vi "Test LockinEngine.vi"(8 "error in (no error)":errorcluster, 11 "Lockin.DAQ":refnum<class "Instrument.DAQ.lvclass">) -> (0 "error out":errorcluster, 3 "Lockin.DAQ":refnum<class "Instrument.DAQ.lvclass">)   [LabVIEW 2019, in "Instrument.Lockin.lvlib" / "Instrument.DAQ.lvclass"]
uses:
  Instrument.DAQ.lvclass
  Typedefs/DAQ.Sampling.Sampling--Cluster.ctl
  <vilib>/Analysis/NI_AALBase.lvlib
  <vilib>/Analysis/baseanly.llb/Mean (DBL).vi
  Instrument.Lockin/Instrument.Lockin.lvclass
  Typedefs/Sweep.State--enum.ctl
  Typedefs/AO.Channel.Function--Enum.ctl
  Typedefs/AO.Channel--Cluster--Array.ctl
  Waveguide Model/Waveguide Model--Cluster.ctl
  Typedefs/AO.Channel--Cluster.ctl
  Typedefs/REF.Channel--Cluster.ctl
  Typedefs/REF.Channel--Cluster--Array.ctl
  Instrument.Lockin/Typedefs/Results Type--Enum.ctl
  Typedefs/AI.Channel--Cluster.ctl
  Typedefs/AI.Channel--Cluster--Array.ctl
panel:
  in  "Configuration.AI Channels":T1 {"References" items=["", "1", "2", "3"]; "Channel" min=1}
  in  "Configuration.Channels: REF":T3 {"Roll-Off" min=1; "TC" min=0.0001 format="%#_3p"; "Phase" format="%.3g"; "Frequency" min=0.0001 max=10000.0 format="%.3g"; "Channel" min=1}
  out "refresh rate (Hz)":dbl
  out "Waveform Graph":dbl[][](graph)
  in  "buffer size (samples)":i32
  in  "intervals":i32=10
  out "Histogram Graph":T5(graph)
  in  "sampling":T6={"Fs"=204789.0, "#s"=15753} {"Fs" format="%#_13g"}
  in  "Type":T7
  in  "stop":bool
  in  "Simulate Waveguide":bool
  out "Average time (ms)":dbl=0.328125
  in  "Waveguide Cluster":T8
  out "Waveform Chart 2":u32(graph)
  out "Waveform Chart":dbl[][](graph)=[[-0.22911635604378638]]
  in  "AO Channels":T9=[{"Enable?"=FALSE, "Channel"=0, "Amplitude"=0.0, "Offset"=0.0, "Frequency"=0.1, "Phase"=0.0, "Function"=enum."Sine", "Sweeping?"=FALSE}] {"Phase" format="%.3g"; "Frequency" min=0.0001 max=10000.0 format="%.3g"; "Offset" format="%.3p"; "Amplitude" min=0.0 max=10.0 format="%.3p"}
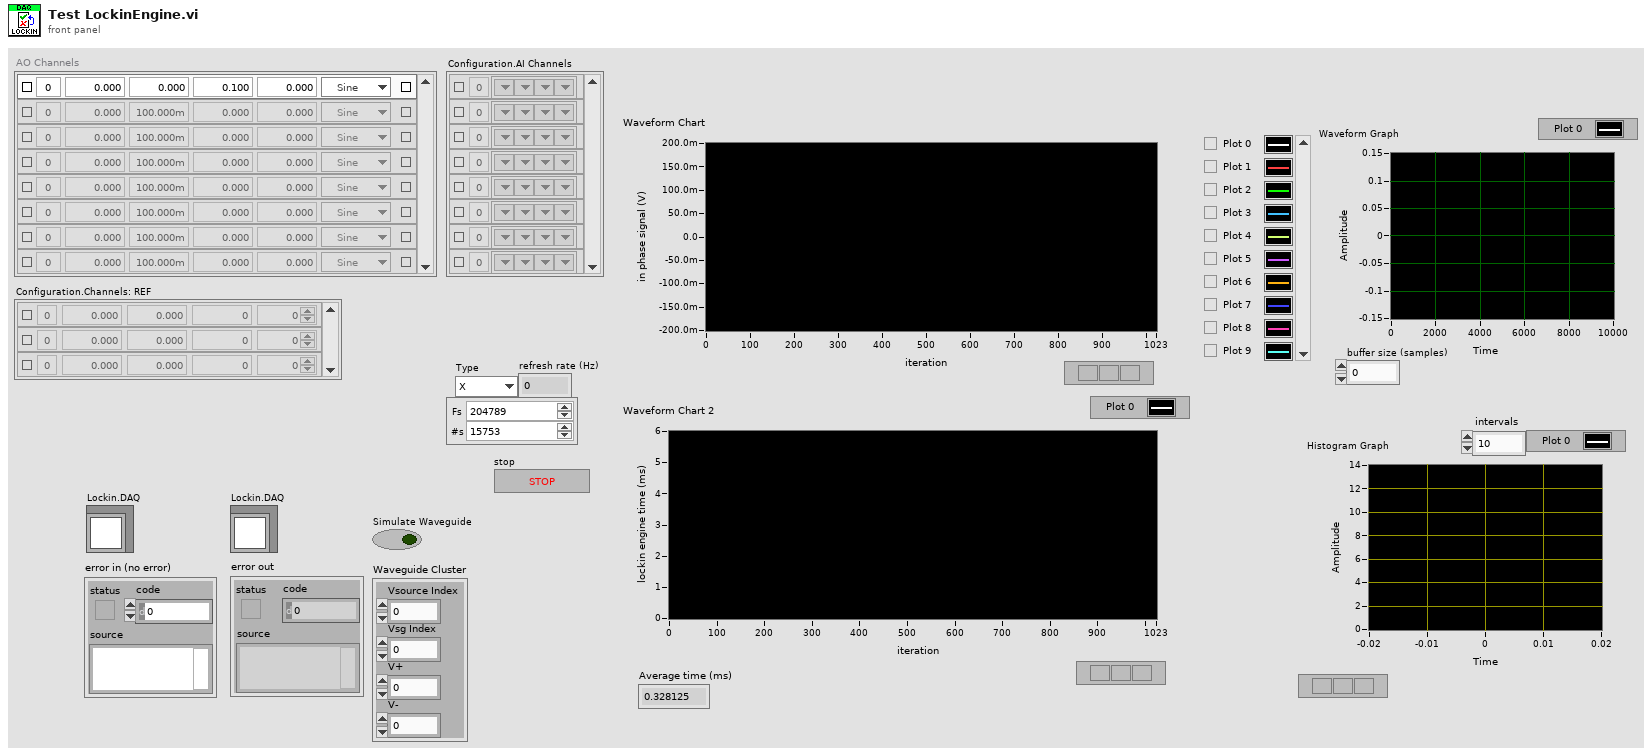
[diagram p1: front panel]
types:
  T1 = typedef "Instrument.Lockin.lvlib/Instrument.DAQ.lvclass/AI.Channel--Cluster--Array.ctl" = T2[]
  T2 = typedef "Instrument.Lockin.lvlib/Instrument.DAQ.lvclass/AI.Channel--Cluster.ctl" = cluster{"Enable?":bool, "Channel":i32, "References":i32[]}
  T3 = typedef "Instrument.Lockin.lvlib/Instrument.DAQ.lvclass/REF.Channel--Cluster--Array.ctl" = T4[]
  T4 = typedef "Instrument.Lockin.lvlib/Instrument.DAQ.lvclass/REF.Channel--Cluster.ctl" = cluster{"Enable?":bool, "Channel":i32, "Frequency":dbl, "Phase":dbl, "TC":dbl, "Roll-Off":i32}
  T5 = cluster{"X Values":dbl[], "Histogram: h(x)":i32[]}[]
  T6 = typedef "Instrument.Lockin.lvlib/Instrument.DAQ.lvclass/DAQ.Sampling.Sampling--Cluster.ctl" = cluster{"Fs":dbl, "#s":i32}
  T7 = typedef "Instrument.Lockin.lvlib/Instrument.Lockin.lvclass/Results Type--Enum.ctl" = enum16{"X", "Y", "R", "Theta", "Mean"}
  T8 = typedef "Instrument.Lockin.lvlib/Instrument.DAQ.lvclass/Waveguide Model--Cluster.ctl" = cluster{"Vsource Index":i32, "Vsg Index":i32, "V+":i32, "V-":i32}
  T9 = typedef "Instrument.Lockin.lvlib/Instrument.DAQ.lvclass/AO.Channel--Cluster--Array.ctl" = T10[]
  T10 = typedef "Instrument.Lockin.lvlib/Instrument.DAQ.lvclass/AO.Channel--Cluster.ctl" = cluster{"Enable?":bool, "Channel":i32, "Amplitude":dbl, "Offset":dbl, "Frequency":dbl, "Phase":dbl, "Function":T11, "Sweeping?":bool}
  T11 = typedef "Instrument.Lockin.lvlib/Instrument.DAQ.lvclass/AO.Channel.Function--Enum.ctl" = enum16{"Sine", "Triangle", "Square"}
  T12 = typedef "Instrument.Lockin.lvlib/Instrument.DAQ.lvclass/Sweep.State--enum.ctl" = enum16{"idle", "initialize", "wait", "sweep", "stop"}
  T13 = typedef "Instrument.Lockin.lvlib/Instrument.DAQ.lvclass/Results--Cluster.ctl" = cluster{"Time Stamp":timestamp, "Results (Dictionary)":cluster{"key":string, "value":dbl}[]}
  T14 = cluster{"X Values":dbl[], "Histogram: h(x)":i32[]}
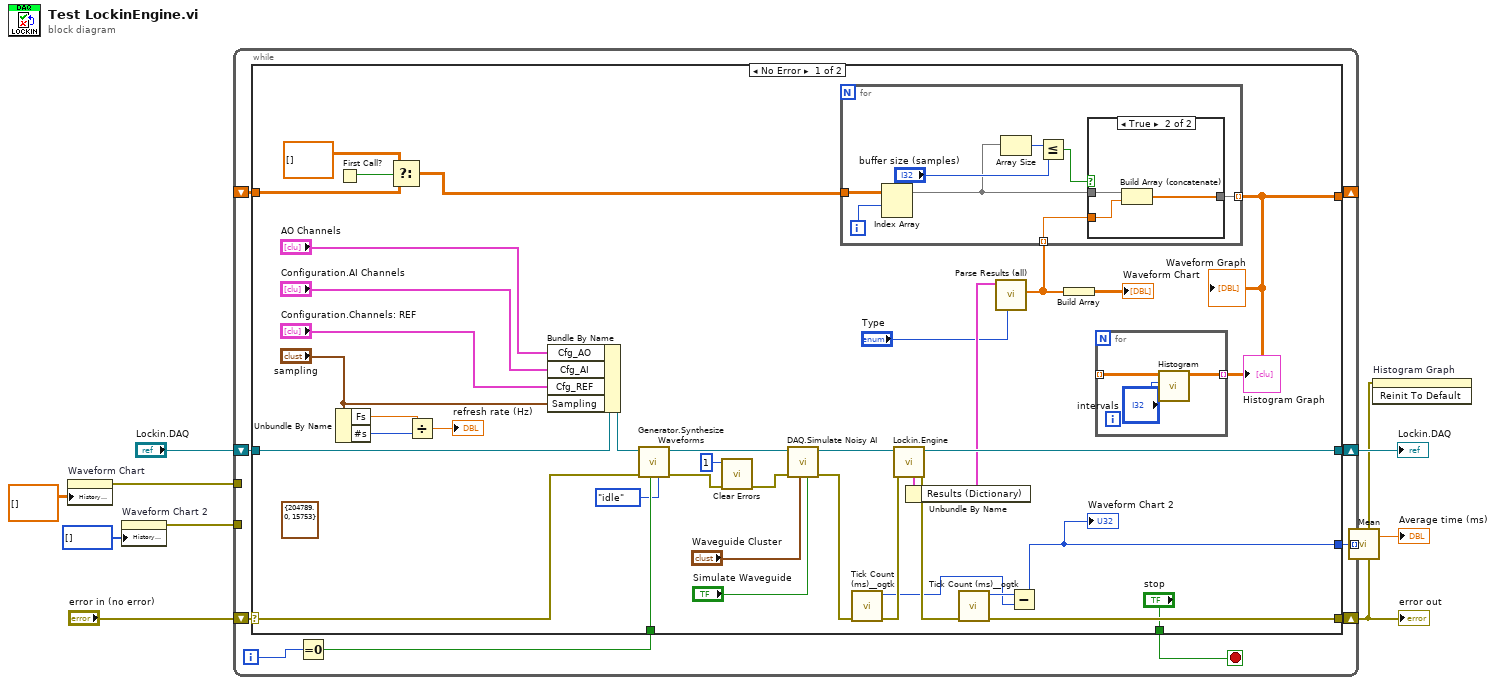
[diagram p0: block diagram]
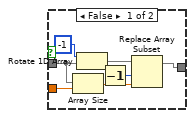
[diagram p2: hidden frame]
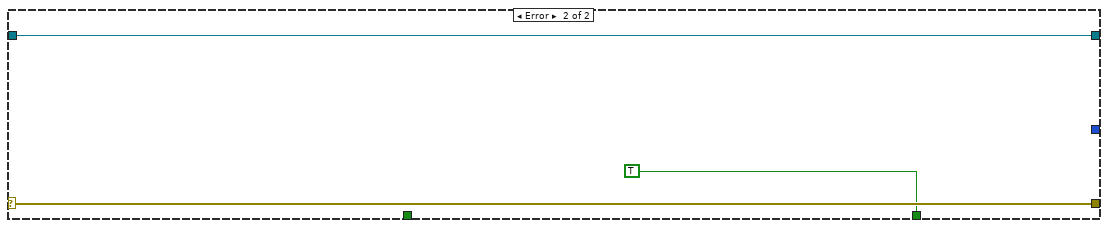
[diagram p3: hidden frame]
diagram:
  n1 = property on="Waveform Chart" class="WFChart (strict)"("History Data"=dbl[][] []) -> (error out=w3:errorcluster)  [unwired: 2 in, 1 out]
  n2 = property on="Waveform Chart 2" class="WFChart (strict)"("History Data"=u32[] []) -> (error out=w4:errorcluster)  [unwired: 2 in, 1 out]
  n3 = while {
    shift-right: [w19] -> w1
    shift-left: "error in (no error)" -> [w20]
    shift-right: [w17] -> w8
    shift-left: "Lockin.DAQ" -> [w18]
    tunnel: [w16] -> w5 mode=indexing
    tunnel: w4 -> [_]
    tunnel: w3 -> [_]
    shift-right: [w12] -> _
    shift-left: _ -> [w11]
    i -> [w14]
    stop <- w13 stop-if-true
    n4 = Equal To 0?(x=w14) -> (x = 0?=w15:bool)
    n5 = case shown="No Error" w20 {
      selector: w20 -> [w58 w83]
      tunnel: [w52 w83] -> w19
      tunnel: [w56 w82] -> w17
      tunnel: w18 -> [w26 w82]
      tunnel: [w50 _] -> w16
      tunnel: w15 -> [w46 _]
      tunnel: ["stop" TRUE ("stop")] -> w13
      tunnel: [w42 _] -> w12
      tunnel: w11 -> [w37 _]
      frame No Error {
        (unwired) T6 {"Fs"=204789.0, "#s"=15753} ("sampling")
        n6 = First Call?() -> (First Call?: T/F=w39:bool)
        n7 = Unbundle By Name("sampling") -> ("Fs"=w36:dbl, "#s"=w35:i32)
        n8 = Select(t=dbl[][] [], s=w39, f=w37) -> (s? t:f=w38:dbl[][])
        n9 = Divide(x=w36, y=w35) -> (x/y=→"refresh rate (Hz)":dbl)
        n10 = Bundle By Name(cluster=w26, "Cfg_AO"="AO Channels", "Cfg_AI"="Configuration.AI Channels", "Cfg_REF"="Configuration.Channels: REF", "Sampling"="sampling") -> (w28:refnum<class "Instrument.DAQ.lvclass">)
        n11 = call "Generator.Synthesize Waveforms.vi"("sweep state"=Sweep.State--enum."idle", "Reset Phase?"=w46, "error in (no error)"=w58, "Instrument.DAQ"=w28) -> ("error out"=w24:errorcluster, "Instrument.DAQ"=w59:refnum<class "Instrument.DAQ.lvclass">)  [unwired: 6 in]
        n12 = call <vilib>:"Clear Errors.vi"("error in (no error)"=w24, "specific error code to clear (0: all)"=1) -> ("error out"=w23:errorcluster)  [unwired: 4 in, 1 out]
        n13 = call "DAQ.Simulate Noisy AI.vi"("Simulate Waveguide [T]"="Simulate Waveguide", "Waveguide Cluster"="Waveguide Cluster", "error in (no error)"=w23, "Instrument.DAQ in"=w59) -> ("error out"=w54:errorcluster, "Instrument.DAQ out"=w57:refnum<class "Instrument.DAQ.lvclass">)  [unwired: 6 in]
        n14 = call <userlib>:"Tick Count (ms)__ogtk.vi"("error in (no error)"=w54) -> ("error out"=w53:errorcluster, "millisecond timer value"=w43:u32)  [unwired: 9 in]
        n15 = call "Lockin.Engine.vi"("error in (no error)"=w53, "Instrument.DAQ"=w57) -> ("error out"=w49:errorcluster, "<Results> (X,Y,R,Theta,Mean)"=w55:T13, "Instrument.DAQ out"=w56:refnum<class "Instrument.DAQ.lvclass">)  [unwired: 7 in]
        n16 = Unbundle By Name(w55) -> ("Results (Dictionary)"=w33:cluster{"key":string, "value":dbl}[])
        n17 = call <userlib>:"Tick Count (ms)__ogtk.vi"("error in (no error)"=w49) -> ("error out"=w52:errorcluster, "millisecond timer value"=w51:u32)  [unwired: 9 in]
        n18 = call "Parse Results (all).vi"("Type"="Type", "Results (Dictionary)"=w33) -> ("Data"=w32:dbl[])  [unwired: 6 in, 3 out]
        n19 = for {
          tunnel: w38 -> [w70]
          tunnel: [w66] -> w42 mode=indexing
          tunnel: w32 -> [w65] mode=indexing
          i -> [w63]
          n20 = Index Array(array=w70, index (row)=w63) -> (element=w64:dbl[])  [unwired: 1 in]
          n21 = Array Size(array=w64) -> (size(s)=w69:i32)
          n22 = Less Or Equal?(x=w69, y="buffer size (samples)") -> (x <= y?=w67:bool)
          n23 = case shown="True" w67 {
            tunnel: [w72 w80] -> w66
            tunnel: w65 -> [w75 w78]
            tunnel: w64 -> [w74 w79]
            frame False {
              n24 = Array Size(array=w74) -> (size(s)=w73:i32)
              n25 = Rotate 1D Array(1:w74, 2:-1 ("n")) -> (0:w76:dbl[])
              n26 = Decrement(x=w73) -> (x-1=w71:i32)
              n27 = Replace Array Subset(array=w76, new element=w75, index=w71) -> (w72:dbl[])
            }
            frame True {
              n28 = Build Array (concatenate)(w79, w78) -> (w80:dbl[])
            }
          }
        }
        "Waveform Graph" <- w42
        n29 = Subtract(x=w51, y=w43) -> (x-y=w50:u32)
        "Waveform Chart 2" <- w50
        n30 = Build Array(w32) -> (→"Waveform Chart":dbl[][])
        n31 = for {
          tunnel: w42 -> [w61] mode=indexing
          tunnel: [w60] -> w41 mode=indexing
          n32 = call <vilib>:"Histogram.vi"("intervals"="intervals", "X"=w61) -> ("Histogram Graph"=w60:T14)  [unwired: 6 in, 3 out]
        }
        "Histogram Graph" <- w41
      }
      frame Error {
      }
    }
  }
  "error out" <- w1
  "Lockin.DAQ" <- w8
  n33 = call-poly <vilib>:"Mean.vi"("X"=w5) -> ("mean"=→"Average time (ms)":dbl)  [unwired: 1 out]
  n34 = invoke on="Histogram Graph" class="XYGraph (strict)" method="Reinit To Default"(error in=w1) -> ()  [unwired: 2 in, 3 out]
